vi "readPress.vi"() -> ()   [LabVIEW 2011]
uses:
  <vilib>/Utility/file.llb/Read From Spreadsheet File (string).vi
panel:
  out "Pressure":string[][](table)
  in  "EXIT":bool
  in  "OK Button":bool
  in  "Boolean":bool caption="Choose date    Today"
  out "Pressure":cluster{dbl[], dbl[]}[](graph)=[{[1.0, 2.0, 4.0], [2.0, 1.0, 0.0]}, {[0.5, 1.5, 3.5], [3.0, 4.0, 2.0]}]
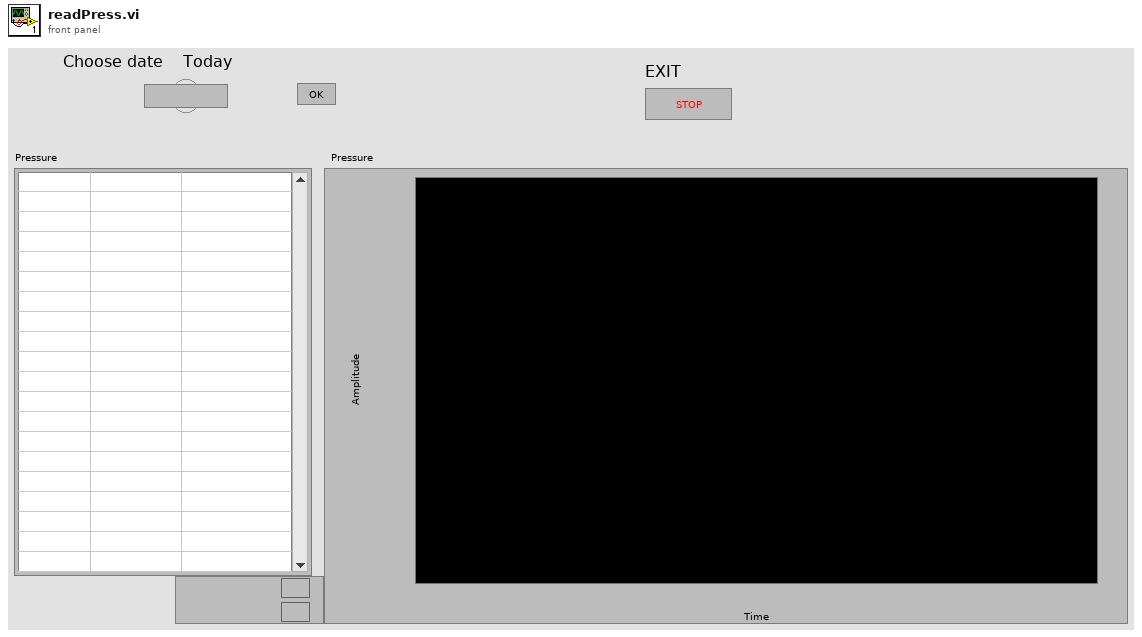
[diagram p1: front panel]
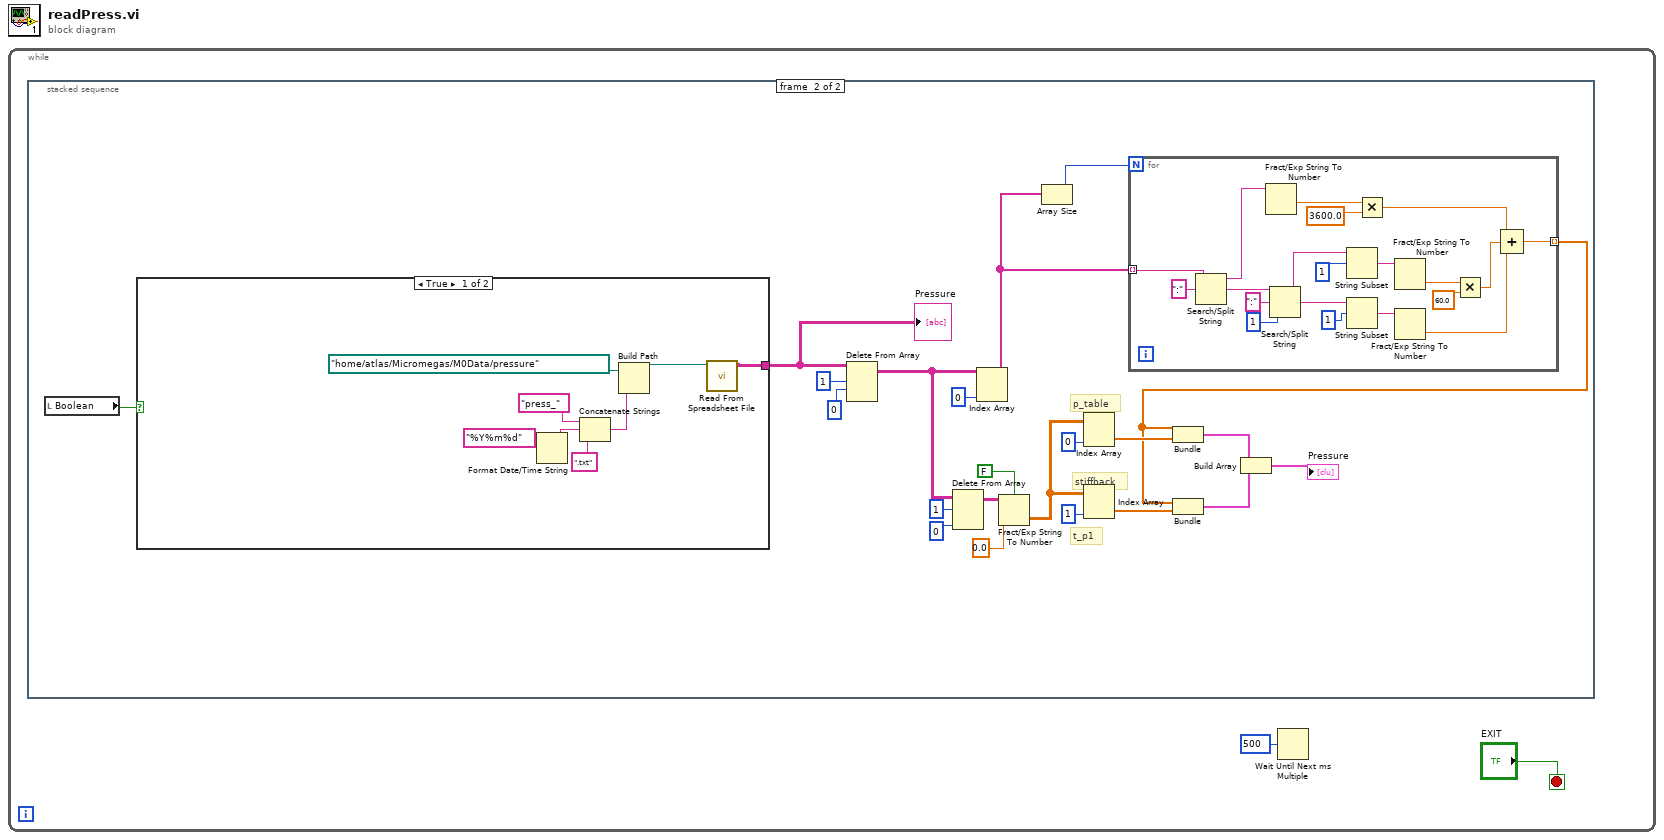
[diagram p0: block diagram]
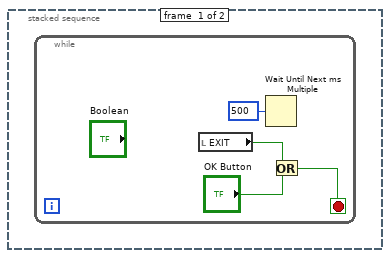
[diagram p2: hidden frame]
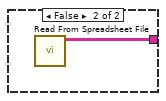
[diagram p3: hidden frame]
diagram:
  n1 = while {
    stop <- "EXIT" stop-if-true
    n2 = stacked-sequence {
      frame #0 {
        n3 = while {
          stop <- w3 stop-if-true
          n4 = local read "EXIT"() -> (w5:bool)
          n5 = Wait Until Next ms Multiple(millisecond multiple=u32 500) -> ()  [unwired: 1 out]
          n6 = Or(x=w5, y="OK Button") -> (x .or. y?=w3:bool)
        }
      }
      frame #1 {
        # "t_p1"
        # "stiffback"
        # "p_table"
        n7 = local read "Boolean"() -> (w9:bool)
        n8 = case shown="True" w9 {
          tunnel: [w31 w37] -> w7
          frame True {
            n9 = Format Date/Time String(time format string (%c)="%Y%m%d") -> (date/time string=w34:string)  [unwired: 2 in]
            n10 = Concatenate Strings("press_" ("string"), w34, ".txt" ("string")) -> (w32:string)
            n11 = Build Path(base path=path "/home/atlas/Micromegas/M0Data/pressure", name or relative path=w32) -> (appended path=w29:path)
            n12 = call-poly <vilib>:"Read From Spreadsheet File.vi"("file path (dialog if empty)"=w29) -> ("all rows"=w31:string[][])  [unwired: 6 in, 4 out]
          }
          frame False {
            n13 = call-poly <vilib>:"Read From Spreadsheet File.vi"() -> ("all rows"=w37:string[][])  [unwired: 7 in, 4 out]
          }
        }
        "Pressure" <- w7
        n14 = Delete From Array(array=w7, length=1, index (row)=0) -> (array with subset deleted=w8:string[][])  [unwired: 1 in, 1 out]
        n15 = Delete From Array(array=w8, length=1, index (col)=0 ("disabled index (col)")) -> (array with subset deleted=w25:string[][])  [unwired: 1 in, 1 out]
        n16 = Index Array(array=w8, index (col)=0 ("disabled index (col)")) -> (element=w23:string[])  [unwired: 1 in]
        n17 = Fract/Exp String To Number(use system decimal point (T)=FALSE, string=w25, default (0 dbl)=0.0 ("default (0 DBL)")) -> (number=w14:dbl[][])  [unwired: 1 in, 1 out]
        n18 = Array Size(array=w23) -> (size(s)=w24:i32)
        n19 = Index Array(array=w14, index (col)=0 ("disabled index (col)")) -> (element=w18:dbl[])  [unwired: 1 in]
        n20 = Index Array(array=w14, index (col)=1 ("disabled index (col)")) -> (element=w17:dbl[])  [unwired: 1 in]
        n21 = for {
          N: w24 -> [_]
          tunnel: w23 -> [w57] mode=indexing
          tunnel: [w49] -> w13 mode=indexing
          n22 = Search/Split String(string=w57, search string/char (-)=":") -> (substring before match=w53:string, match + rest of string=w54:string)  [unwired: 1 in, 1 out]
          n23 = Fract/Exp String To Number(string=w53) -> (number=w41:dbl)  [unwired: 3 in, 1 out]
          n24 = Search/Split String(string=w54, search string/char (-)=":", offset (0)=1) -> (substring before match=w47:string, match + rest of string=w43:string)  [unwired: 1 out]
          n25 = String Subset(string=w47, offset (0)=1) -> (substring=w45:string)  [unwired: 1 in]
          n26 = String Subset(string=w43, offset (0)=1) -> (substring=w42:string)  [unwired: 1 in]
          n27 = Multiply(x=w41, y=3600.0) -> (x*y=w40:dbl)
          n28 = Fract/Exp String To Number(string=w45) -> (number=w50:dbl)  [unwired: 3 in, 1 out]
          n29 = Fract/Exp String To Number(string=w42) -> (number=w38:dbl)  [unwired: 3 in, 1 out]
          n30 = Multiply(x=w50, y=60.0) -> (x*y=w39:dbl)
          n31 = Compound Arithmetic op=ADD(w40, w39, w38) -> (w49:dbl)
        }
        n32 = Bundle(w13, w18) -> (w12:cluster{dbl[], dbl[]})  [unwired: 1 in]
        n33 = Bundle(w13, w17) -> (w11:cluster{dbl[], dbl[]})  [unwired: 1 in]
        n34 = Build Array(w12, w11) -> (→"Pressure":cluster{dbl[], dbl[]}[])
      }
    }
    n35 = Wait Until Next ms Multiple(millisecond multiple=u32 500) -> ()  [unwired: 1 out]
  }
